vi "Setup Memory.vi"(4 "Template Waveform (0: Sine)":i32(ring) items=["Sine", "Square", "Pulse", "Ramp", "Noise"], 5 "Target Memory (0: User 1)":i32(ring) items=["User 1", "User 2", "User 3", "User 4", "Edit Memory", "Edit Memory 1", "Edit Memory 2"], 6 "Point Number (1000)":i32=1000, 7 "Source Memory (4: Edit Memory)":i32(ring)=4 items=["User 1", "User 2", "User 3", "User 4", "Edit Memory", "Edit Memory 1", "Edit Memory 2"], 8 "error in (no error)":errorcluster, 9 "Reset Memory Option (0: Default Setting)":i32(ring) items=["Default Setting", "Set Point Number", "Template Setting"], 10 "Operation Select (0: List Memory)":i32(ring) items=["List Memory", "Copy Memory", "Copy Edit Memory", "Reset Memory"], 11 "VISA resource name":refnum<visa-resource-name>) -> (0 "error out":errorcluster, 2 "Memory List":string, 3 "VISA resource name out":refnum<visa-resource-name>)   [LabVIEW 2015, in "Tektronix AFG 3000 Series.lvlib"]
doc: "Resets, copies or lists memory waveforms.\n\n<B>Note:</B>\n \nThis VI is only applicable for AFG 3KC series."
uses:
  Tektronix AFG 3000 Series.lvlib
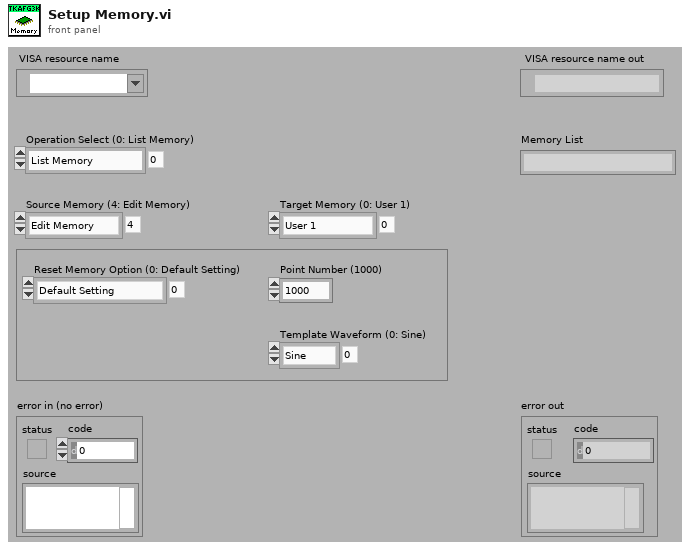
[diagram p1: front panel]
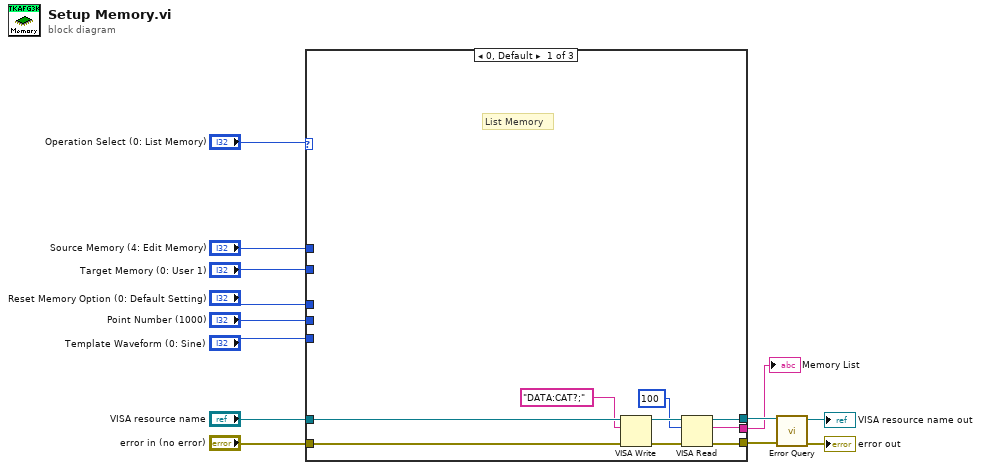
[diagram p0: block diagram]
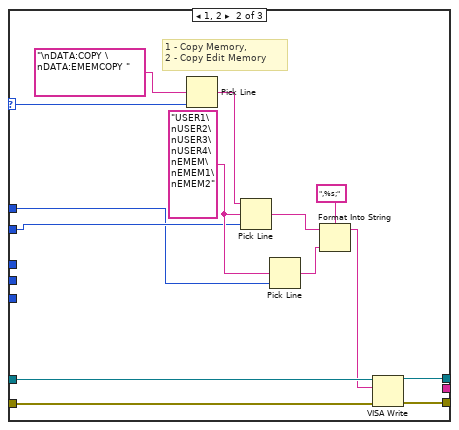
[diagram p2: hidden frame]
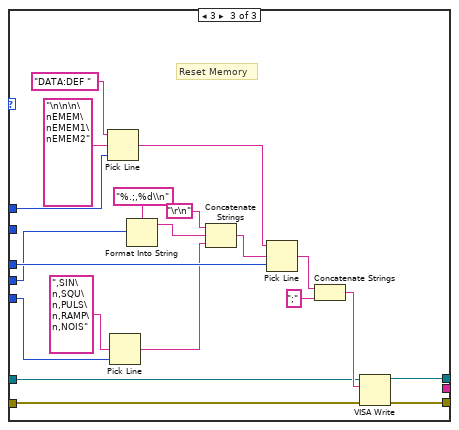
[diagram p3: hidden frame]
diagram:
  n1 = case shown="0, Default" "Operation Select (0: List Memory)" {
    selector: "Operation Select (0: List Memory)" -> [_ w32 _]
    tunnel: "Source Memory (4: Edit Memory)" -> [_ w23 w54]
    tunnel: "Target Memory (0: User 1)" -> [_ w24 _]
    tunnel: "Reset Memory Option (0: Default Setting)" -> [_ _ w53]
    tunnel: "Point Number (1000)" -> [_ _ w48]
    tunnel: "Template Waveform (0: Sine)" -> [_ _ w51]
    tunnel: "VISA resource name" -> [w22 w29 w40]
    tunnel: "error in (no error)" -> [w21 w28 w39]
    tunnel: [w16 w26 w38] -> w3
    tunnel: [w17 w25 w37] -> w2
    tunnel: [w15 _ _] -> w1
    frame 0, Default {
      # "List Memory"
      n2 = VISA Write(VISA resource name=w22, write buffer="DATA:CAT?;" ("string (\"\")"), error in (no error)=w21) -> (VISA resource name out=w19:refnum<visa-resource-name>, error out=w18:errorcluster)  [unwired: 1 out]
      n3 = VISA Read(VISA resource name=w19, byte count=u32 100, error in (no error)=w18) -> (VISA resource name out=w16:refnum<visa-resource-name>, read buffer=w15:string, error out=w17:errorcluster)  [unwired: 1 out]
    }
    frame 1, 2 {
      w35 = "USER1\nUSER2\nUSER3\nUSER4\nEMEM\nEMEM1\nEMEM2" ("string (\"\")")
      # "1 - Copy Memory,\n2 - Copy Edit Memory"
      n4 = Pick Line(multi-line string="\nDATA:COPY \nDATA:EMEMCOPY " ("string (\"\")"), line index=w32) -> (output string=w30:string)  [unwired: 1 in]
      n5 = Pick Line(string ("")=w30, multi-line string=w35, line index=w24) -> (output string=w34:string)
      n6 = Pick Line(multi-line string=w35, line index=w23) -> (output string=w33:string)  [unwired: 1 in]
      n7 = Format Into String(format string=",%s;", initial string=w34, w33) -> (resulting string=w27:string)  [unwired: 1 in, 1 out]
      n8 = VISA Write(VISA resource name=w29, write buffer=w27, error in (no error)=w28) -> (VISA resource name out=w26:refnum<visa-resource-name>, error out=w25:errorcluster)  [unwired: 1 out]
    }
    frame 3 {
      # "Reset Memory"
      n9 = Pick Line(string ("")="DATA:DEF ", multi-line string="\n\n\n\nEMEM\nEMEM1\nEMEM2" ("string (\"\")"), line index=w54) -> (output string=w52:string)
      n10 = Pick Line(multi-line string=",SIN\n,SQU\n,PULS\n,RAMP\n,NOIS" ("string (\"\")"), line index=w51) -> (output string=w46:string)  [unwired: 1 in]
      n11 = Format Into String(format string="%.;,%d\\n" ("string (\"\")"), w48) -> (resulting string=w47:string)  [unwired: 2 in, 1 out]
      n12 = Concatenate Strings("\r\n", w47, w46) -> (w44:string)
      n13 = Pick Line(string ("")=w52, multi-line string=w44, line index=w53) -> (output string=w43:string)
      n14 = Concatenate Strings(w43, ";" ("string")) -> (w41:string)
      n15 = VISA Write(VISA resource name=w40, write buffer=w41, error in (no error)=w39) -> (VISA resource name out=w38:refnum<visa-resource-name>, error out=w37:errorcluster)  [unwired: 1 out]
    }
  }
  "Memory List" <- w1
  n16 = call "Error Query.vi"("error in (no error)"=w2, "VISA resource name"=w3) -> ("error out"=→"error out":errorcluster, "VISA resource name out"=→"VISA resource name out":refnum<visa-resource-name>)  [unwired: 6 in, 2 out]
